vi "AO Update.vi"(8 "error in (no error)":errorcluster, 11 "Simple Analog Output in":refnum<class "Simple Analog Output.lvclass">) -> (0 "error out":errorcluster, 3 "Simple Analog Output out":refnum<class "Simple Analog Output.lvclass">)   [LabVIEW 2020, in "Instrument.lvlib" / "Simple Analog Output.lvclass"]
uses:
  Simple Analog Output.lvclass
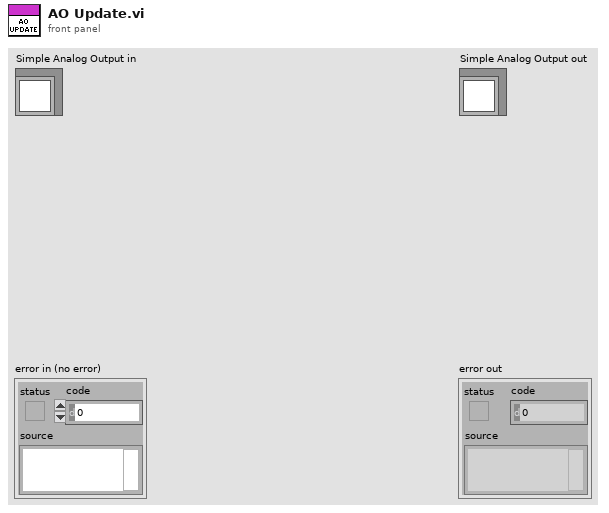
[diagram p1: front panel]
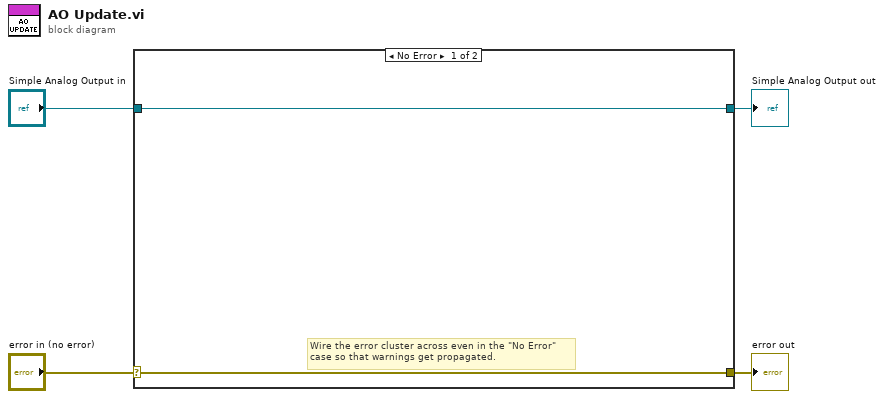
[diagram p0: block diagram]
diagram:
  n1 = case shown="No Error" "error in (no error)" {
    selector: "error in (no error)" -> [w5 w8]
    tunnel: [w5 w8] -> w3
    tunnel: [w6 w7] -> w1
    tunnel: "Simple Analog Output in" -> [w6 w7]
    frame No Error {
      # "Wire the error cluster across even in the \"No Error\"\ncase so that warnings get propagated."
    }
    frame Error {
    }
  }
  "error out" <- w3
  "Simple Analog Output out" <- w1
